vi "DriveArcadeMixer.vi"(10 "X axis (turning) value":dbl, 11 "Y axis (throttle) value":dbl) -> (2 "Right Motor Value":dbl, 3 "Left Motor Value":dbl)   [LabVIEW 2017]
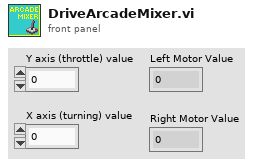
[diagram p1: front panel]
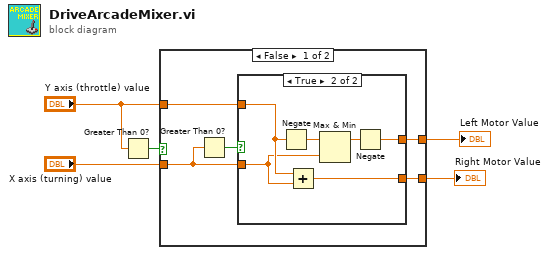
[diagram p0: block diagram]
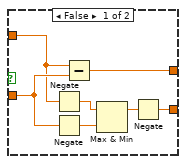
[diagram p2: hidden frame]
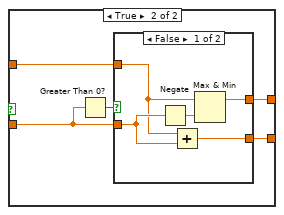
[diagram p3: hidden frame]
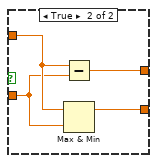
[diagram p4: hidden frame]
diagram:
  n1 = Greater Than 0?(x="Y axis (throttle) value") -> (x > 0?=w1:bool)
  n2 = case shown="False" w1 {
    tunnel: "X axis (turning) value" -> [w9 w27]
    tunnel: "Y axis (throttle) value" -> [w8 w26]
    tunnel: [w7 w25] -> w4
    tunnel: [w6 w24] -> w5
    frame False {
      n3 = Greater Than 0?(x=w9) -> (x > 0?=w10:bool)
      n4 = case shown="True" w10 {
        tunnel: w9 -> [w17 w19]
        tunnel: w8 -> [w15 w20]
        tunnel: [w11 w21] -> w7
        tunnel: [w12 w18] -> w6
        frame False {
          n5 = Negate(x=w15) -> (-x=w16:dbl)
          n6 = Negate(x=w17) -> (-x=w14:dbl)
          n7 = Subtract(x=w15, y=w17) -> (x-y=w11:dbl)
          n8 = Max & Min(x=w16, y=w14) -> (max(x,y)=w13:dbl)  [unwired: 1 out]
          n9 = Negate(x=w13) -> (-x=w12:dbl)
        }
        frame True {
          n10 = Negate(x=w20) -> (-x=w23:dbl)
          n11 = Add(x=w20, y=w19) -> (x+y=w18:dbl)
          n12 = Max & Min(x=w23, y=w19) -> (max(x,y)=w22:dbl)  [unwired: 1 out]
          n13 = Negate(x=w22) -> (-x=w21:dbl)
        }
      }
    }
    frame True {
      n14 = Greater Than 0?(x=w27) -> (x > 0?=w28:bool)
      n15 = case shown="False" w28 {
        tunnel: w27 -> [w33 w35]
        tunnel: w26 -> [w30 w36]
        tunnel: [w31 w34] -> w25
        tunnel: [w29 w37] -> w24
        frame False {
          n16 = Negate(x=w33) -> (-x=w32:dbl)
          n17 = Add(x=w30, y=w33) -> (x+y=w29:dbl)
          n18 = Max & Min(x=w30, y=w32) -> (max(x,y)=w31:dbl)  [unwired: 1 out]
        }
        frame True {
          n19 = Subtract(x=w36, y=w35) -> (x-y=w34:dbl)
          n20 = Max & Min(x=w36, y=w35) -> (max(x,y)=w37:dbl)  [unwired: 1 out]
        }
      }
    }
  }
  "Right Motor Value" <- w5
  "Left Motor Value" <- w4
